vi "Add Device.vi"(8 "error in (no error)":errorcluster, 11 "Configuration UI in":refnum<class "Configuration UI.lvclass">) -> (0 "error out":errorcluster, 3 "Configuration UI out":refnum<class "Configuration UI.lvclass">)   [LabVIEW 2019, in "Configuration UI.lvlib" / "Configuration UI.lvclass"]
doc: "This routine \n1. Prompts the user to select a device to add to the configuration by calling <b>Config:New Device Dialog</b>\n2. Loads the required keys by calling <b>Load Required Keys</b> \n3. Updates the GUI to show the required configuration keys by calling <b>Refresh Display</b> \n4. Saves the new record to config.ini by calling <b>Save Keys</b> \n5. Calls <b>Select Instrument</b>, choosing the new device to ensure that the config.ini file has been updated with the new record\n6. Calls <b>Engine:Check for Error</b> to confirm no errors occurred."
uses:
  Project/Configuration UI.lvclass
  C:/Users/Public/Documents/Development/builds/Engine/Engine.lvlibp/Project/Engine.lvclass
  Project/Configuration UI.lvclass/Configuration UI.ctl
  Configuration UI Messages/Select Instrument Msg/Select Instrument Msg.lvclass/Select Instrument Msg.ctl
  Accessors/Read Instrument Listbox.vi
  builds/Engine/Engine.lvlibp/Accessors/Read Self Q.vi
  builds/Engine/Actor Framework.lvlibp/1abvi3w/vi.lib/ActorFramework/Message Enqueuer/Enqueue.vi
  builds/Engine/Actor Framework.lvlibp/1abvi3w/vi.lib/ActorFramework/Message Enqueuer/Message Enqueuer.lvclass
  Configuration UI Messages/Select Instrument Msg/Select Instrument Msg.lvclass
  builds/Tools/Config.lvlibp/Config.lvclass
  builds/Engine/Engine.lvlibp/Project/Engine.lvclass
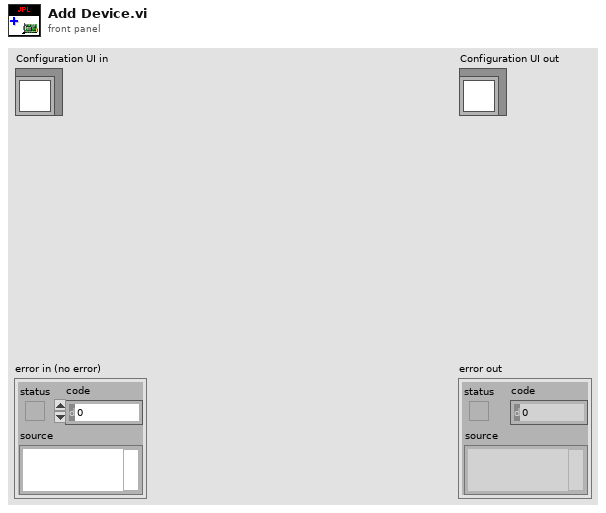
[diagram p1: front panel]
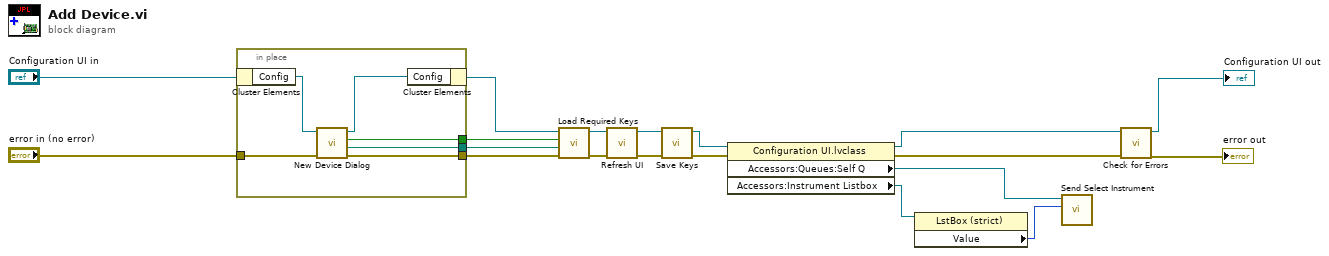
[diagram p0: block diagram]
diagram:
  n1 = in-place {
    in-place-border: "error in (no error)" -> [w23]
    in-place-border: [w22] -> w16
    in-place-border: [w21] -> w14
    in-place-border: [w20] -> w15
    n2 = in-place-cluster #1("Configuration UI in") -> ("Config"=w25:refnum<class "Config.lvclass">)
    n3 = call "New Device Dialog.vi"("error in"=w23, "Config in"=w25) -> ("error out"=w22:errorcluster, "Class Path"=w21:path, "Cancelled"=w20:bool, "Config out"=w24:refnum<class "Config.lvclass">)  [unwired: 6 in]
    n4 = in-place-cluster #1("Config"=w24) -> (w17:refnum<class "Configuration UI.lvclass">)
  }
  n5 = call "Load Required Keys.vi"("error in"=w16, "Class Path"=w14, "Cancelled"=w15, "Configuration UI in"=w17) -> ("error out"=w10:errorcluster, "Configuration UI out"=w11:refnum<class "Configuration UI.lvclass">)  [unwired: 6 in]
  n6 = call "Refresh UI.vi"("error in (no error)"=w10, "Configuration UI in"=w11) -> ("error out"=w4:errorcluster, "Configuration UI out"=w3:refnum<class "Configuration UI.lvclass">)  [unwired: 8 in]
  n7 = call "Save Keys.vi"("error in (no error)"=w4, "Configuration UI in"=w3) -> ("error out"=w1:errorcluster, "Configuration UI out"=w2:refnum<class "Configuration UI.lvclass">)  [unwired: 8 in]
  n8 = property class="Configuration UI.lvclass"(reference=w2, error in=w1) -> (reference out=w6:refnum<class "Configuration UI.lvclass">, error out=w5:errorcluster, "Accessors:Queues:Self Q"=w9:refnum<class "Message Enqueuer.lvclass">, "Accessors:Instrument Listbox"=w8:refnum<vi>)
  n9 = property class="LstBox (strict)"(reference=w8) -> ("Value"=w7:i32)  [unwired: 1 in, 2 out]
  n10 = call "Send Select Instrument.vi"("Selected"=w7, "Message Enqueuer"=w9) -> ()  [unwired: 8 in, 2 out]
  n11 = call "Check for Errors.vi"("error in"=w5, "Engine in"=w6) -> ("error out"=→"error out":errorcluster, "Engine out"=→"Configuration UI out":refnum<class "Configuration UI.lvclass">)  [unwired: 8 in]
